vi "Subset Transfer Data from Group.vi"(5 "transfer id":i32, 7 "transfer group id":i32, 8 "error in (no error)":errorcluster, 10 "group data in":string, 11 "UDP Transceiver in":refnum<class "UDP Transceiver.lvclass">) -> (0 "error out":errorcluster, 1 "transfer data":string, 2 "group data out":string, 3 "UDP Transceiver out":refnum<class "UDP Transceiver.lvclass">)   [LabVIEW 2017, in "UDP Transceiver.lvlib" / "UDP Transceiver.lvclass"]
uses:
  UDP Transceiver.lvclass
  UDP Transceiver.lvclass/UDP Transceiver.ctl
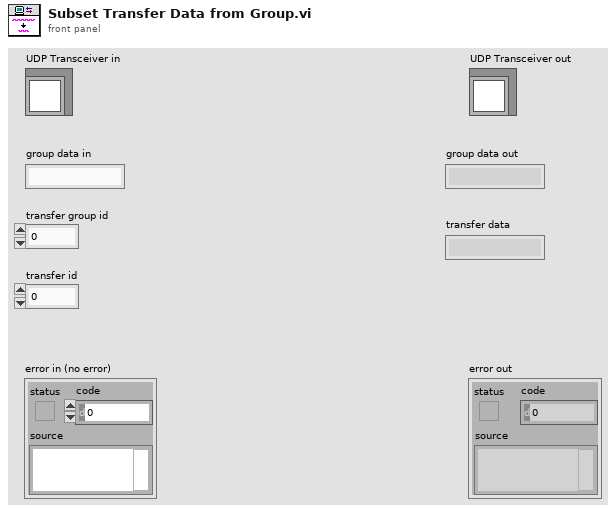
[diagram p1: front panel]
types:
  T1 = typedef "UDP Transceiver.lvlib/UDP Transceiver.lvclass/Transfer Group Parameters.ctl" = cluster{"transfers":T2[], "max size":i32, "timeout":i32}
  T2 = typedef "UDP Transceiver.lvlib/UDP Transceiver.lvclass/Transfer Parameters.ctl" = cluster{"group offset":u64, "size":u64, "address":u32, "port":u16}
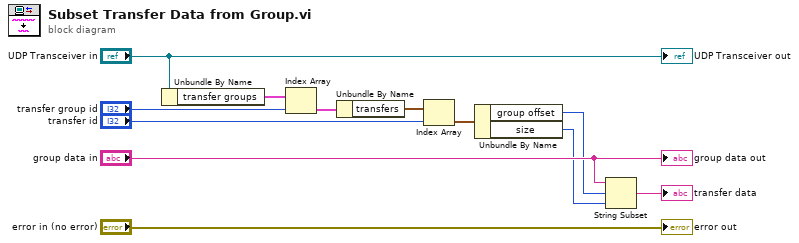
[diagram p0: block diagram]
diagram:
  n1 = Unbundle By Name("UDP Transceiver in") -> ("transfer groups"=w11:T1[])
  n2 = Index Array(array=w11, index="transfer group id") -> (element=w10:T1)
  n3 = Unbundle By Name(w10) -> ("transfers"=w8:T2[])
  n4 = Index Array(array=w8, index="transfer id") -> (element=w9:T2)
  n5 = Unbundle By Name(w9) -> ("group offset"=w2:u64, "size"=w3:u64)
  n6 = String Subset(string="group data in", offset (0)=w2, length (rest)=w3) -> (substring=→"transfer data":string)
  "error out" <- "error in (no error)"
  "UDP Transceiver out" <- "UDP Transceiver in"
  "group data out" <- "group data in"
